vi "TimerCalc state.vi"(8 "error in (no error)":errorcluster, 10 "GUI":refnum<queue>, 11 "Data Cluster in":T1) -> (0 "error out":errorcluster, 3 "Data Cluster out":T1)   [LabVIEW 2015]
uses:
  controls/UI Data.ctl
  DatabaseManager/DBManager.lvclass
  support/Message Queue/Message Cluster.ctl
  <vilib>/Utility/miscctls.llb/LVDateTimeRec.ctl
  support/Message Queue/Enqueue Message (Single).vi
  support/Message Queue/Message Queue.lvlib
panel:
  # "Connector Pane"
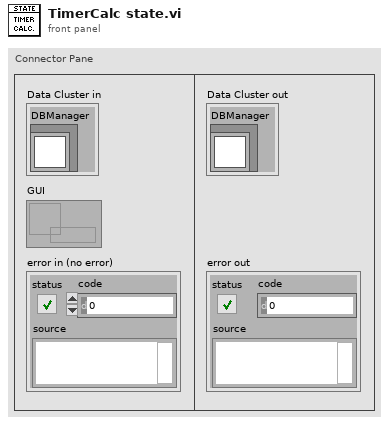
[diagram p1: front panel]
types:
  T1 = typedef "UI Data.ctl" = cluster{"DBManager":refnum<class "DBManager.lvclass">}
  T2 = typedef "LVDateTimeRec.ctl" = cluster{"fractional second":dbl, "second":i32, "minute":i32, "hour":i32, "day of month":i32, "month":i32, "year":i32, "day of week":i32, "day of year":i32, "DST":i32}
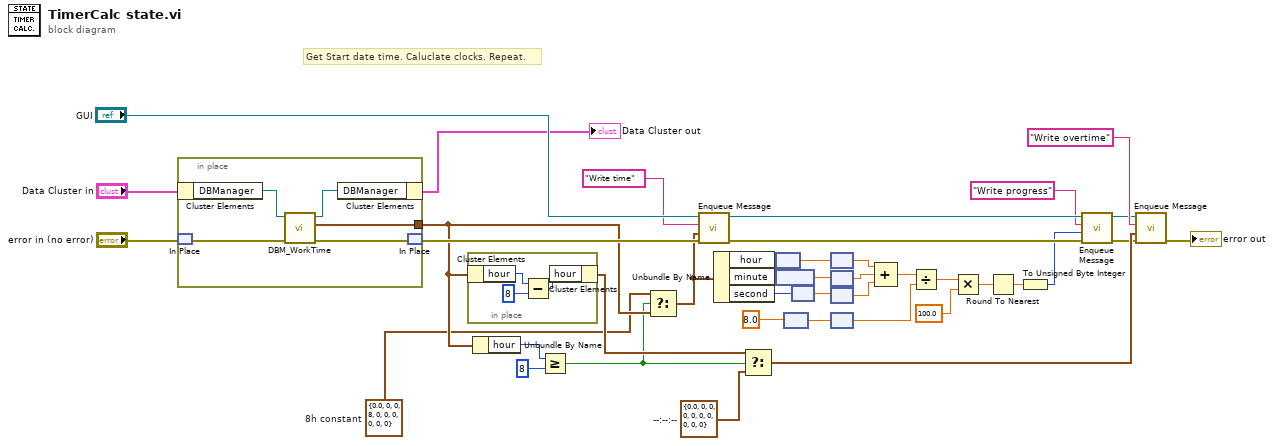
[diagram p0: block diagram]
diagram:
  w26 = T2 {"fractional second"=0.0, "second"=0, "minute"=0, "hour"=8, "day of month"=0, "month"=0, "year"=0, "day of week"=0, "day of year"=0, "DST"=0}  # 8h constant
  w30 = T2 {"fractional second"=0.0, "second"=0, "minute"=0, "hour"=0, "day of month"=0, "month"=0, "year"=0, "day of week"=0, "day of year"=0, "DST"=0}  # --:--:--
  # "Get Start date time. Caluclate clocks. Repeat."
  n1 = in-place {
    in-place-border: [w41] -> w27
    n2 = in-place-cluster #1("Data Cluster in") -> ("DBManager"=w45:refnum<class "DBManager.lvclass">)
    n3 = in-place-match #2("error in (no error)") -> (w44:errorcluster)
    n4 = call "DBM_WorkTime.vi"("error in (no error)"=w44, "DBManager in"=w45) -> ("error out"=w42:errorcluster, "date time rec"=w41:T2, "DBManager out"=w43:refnum<class "DBManager.lvclass">)  [unwired: 7 in]
    n5 = in-place-cluster #1("DBManager"=w43) -> (→"Data Cluster out":T1)
    n6 = in-place-match #2(w42) -> (w38:errorcluster)
  }
  n7 = in-place {
    n8 = in-place-cluster #3(w27) -> ("hour"=w48:i32)
    n9 = Subtract(x=w48, y=8) -> (x-y=w46:i32)
    n10 = in-place-cluster #3("hour"=w46) -> (w29:T2)
  }
  n11 = Unbundle By Name(w27) -> ("hour"=w32:i32)
  n12 = Greater Or Equal?(x=w32, y=8) -> (x >= y?=w25:bool)
  n13 = Select(t=w26, s=w25, f=w27) -> (s? t:f=w20:T2)
  n14 = call-poly "Enqueue Message.vi"("error in (no error)"=w38, "Message Data"=w20, "Message"="Write time", "Message Queue"="GUI") -> ("error out"=w23:errorcluster, "dup Message Queue"=w24:refnum<queue>)  [unwired: 6 in]
  n15 = Unbundle By Name(w20) -> ("hour"=w19:i32, "minute"=w18:i32, "second"=w17:i32)
  n16 = Select(t=w29, s=w25, f=w30) -> (s? t:f=w28:T2)
  n17 = node(w19) -> (w16:dbl[unit])
  n18 = node(w18) -> (w13:dbl[unit])
  n19 = node(8.0) -> (w9:dbl[unit])
  n20 = node(w17) -> (w12:dbl[unit])
  n21 = node(w16) -> (w15:dbl)
  n22 = node(w13) -> (w14:dbl)
  n23 = node(w12) -> (w11:dbl)
  n24 = node(w9) -> (w7:dbl)
  n25 = Compound Arithmetic op=ADD(w15, w14, w11) -> (w8:dbl)
  n26 = Divide(x=w8, y=w7) -> (x/y=w6:dbl)
  n27 = Multiply(x=w6, y=100.0) -> (x*y=w4:dbl)
  n28 = Round To Nearest(number=w4) -> (nearest integer value=w3:dbl)
  n29 = To Unsigned Byte Integer(number=w3) -> (unsigned 8bit integer=w2:u8)
  n30 = call-poly "Enqueue Message.vi"("error in (no error)"=w23, "Message Data"=w2, "Message"="Write progress", "Message Queue"=w24) -> ("error out"=w21:errorcluster, "dup Message Queue"=w22:refnum<queue>)  [unwired: 6 in]
  n31 = call-poly "Enqueue Message.vi"("error in (no error)"=w21, "Message Data"=w28, "Message"="Write overtime", "Message Queue"=w22) -> ("error out"=→"error out":errorcluster)  [unwired: 6 in, 1 out]
